vi "LoadFromText.vi"(8 "error in":errorcluster, 9 "String":string, 10 "editor refs":refnum<vi>[](array[refnum]), 11 "Tree ref":refnum<vi>) -> (0 "error out":errorcluster, 3 "Tree ref out":refnum<vi>)   [LabVIEW 2019, in "ScriptManager.lvlib"]
uses:
  ScriptManager.lvlib
  <vilib>/regexp/Match Regular Expression.xnode
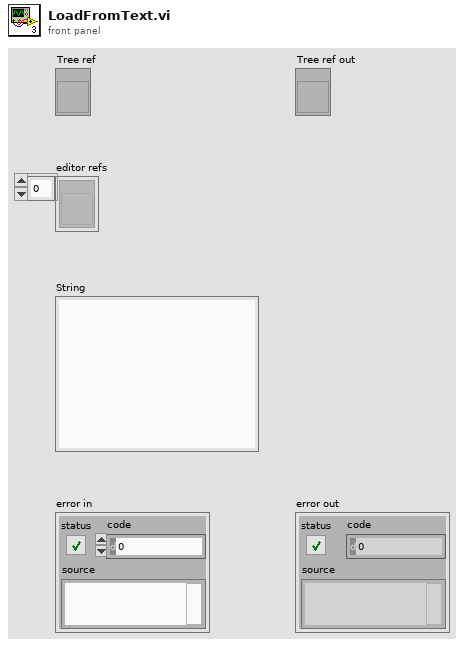
[diagram p1: front panel]
types:
  T1 = cluster{"Left Cell String":string, "Child Text":string[], "Item Indent":i32, "Open?":bool, "Symbol":i32}
  T2 = cluster{"[0]":string, "[1]":string, "[2]":string, "[3]":string, "[4]":string, "[5]":string, "[6]":string, "[7]":string}
  T3 = cluster{"[0]":i32, "[1]":i32, "[2]":i32, "[3]":i32}
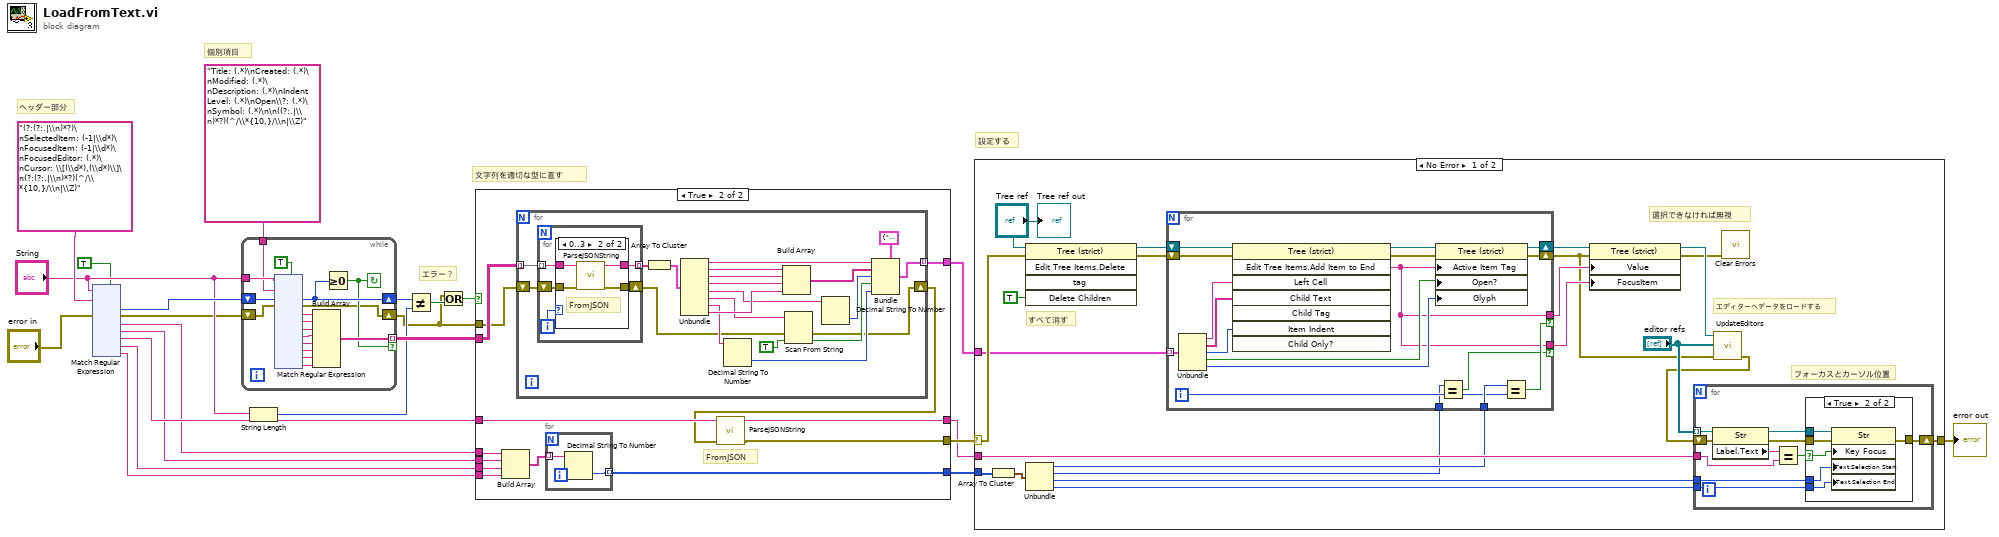
[diagram p0: block diagram]
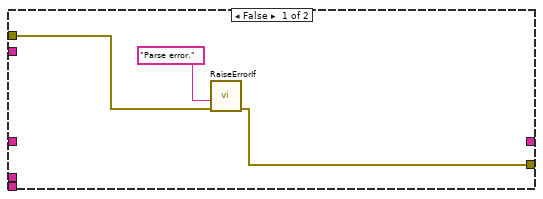
[diagram p4: hidden frame]
diagram:
  # "設定する"
  # "文字列を適切な型に直す"
  # "エラー？"
  # "ヘッダー部分"
  # "個別項目"
  n1 = xnode "Match Regular Expression"("input string"="String", "regular expression"="(?:(?:.|\\n)*?)\nSelectedItem: (-1|\\d*)\nFocusedItem: (-1|\\d*)\nFocusedEditor: (.*)\nCursor: \\[(\\d*),(\\d*)\\]\n(?:(?:.|\\n)*?)(^/\\*{10,}/\\n|\\Z)", "error in"="error in", "multiline? (F)"=TRUE) -> ("offset past match"=w21:i32, "error out"=w14:errorcluster, "submatch 1"=w1:string, "submatch 2"=w2:string, "submatch 3"=w3:string, "submatch 4"=w4:string, "submatch 5"=w5:string)  [unwired: 2 in, 3 out]
  n2 = while {
    tunnel: "String" -> [w40]
    tunnel: "Title: (.*)\nCreated: (.*)\nModified: (.*)\nDescription: (.*)\nIndent Level: (.*)\nOpen\\?: (.*)\nSymbol: (.*)\n\n((?:.|\\n)*?)(^/\\*{10,}/\\n|\\Z)" ("regular expression") -> [w39]
    shift-right: [w36] -> w18
    shift-left: w21 -> [w37]
    tunnel: [w27] -> w22 mode=indexing if=w26
    shift-right: [w24] -> w12
    shift-left: w14 -> [w25]
    stop <- w26 continue-if-true
    n3 = xnode "Match Regular Expression"("input string"=w40, "regular expression"=w39, "offset (0)"=w37, "error in"=w25, "multiline? (F)"=TRUE) -> ("offset past match"=w36:i32, "error out"=w24:errorcluster, "submatch 1"=w35:string, "submatch 2"=w34:string, "submatch 3"=w33:string, "submatch 4"=w32:string, "submatch 5"=w31:string, "submatch 6"=w30:string, "submatch 7"=w29:string, "submatch 8"=w28:string)  [unwired: 1 in, 3 out]
    n4 = Build Array(w35, w34, w33, w32, w31, w30, w29, w28) -> (w27:string[])
    n5 = Greater Or Equal To 0?(x=w36) -> (x >= 0?=w26:bool)
  }
  n6 = String Length(string="String") -> (length=w17:i32)
  n7 = Not Equal?(x=w18, y=w17) -> (x != y?=w16:bool)
  n8 = Or(x=w12, y=w16) -> (x .or. y?=w13:bool)
  n9 = case shown="True" w13 {
    tunnel: w22 -> [_ w182]
    tunnel: w12 -> [w167 w181]
    tunnel: w2 -> [_ w180]
    tunnel: w3 -> [_ w177]
    tunnel: w4 -> [_ w179]
    tunnel: w5 -> [_ w178]
    tunnel: [_ w175] -> w9
    tunnel: [w168 w173] -> w11
    tunnel: [_ w172] -> w8
    tunnel: [_ w171] -> w10
    tunnel: w1 -> [_ w170]
    frame False {
      n10 = call "RaiseErrorIf.vi"("error in (no error)"=w167, "error message"="Parse error.") -> ("error out"=w168:errorcluster)  [unwired: 9 in]
    }
    frame True {
      # "FromJSON"
      n11 = Build Array(w170, w180, w179, w178) -> (w176:string[])
      n12 = for {
        tunnel: w182 -> [w204] mode=indexing
        shift-right: [w186] -> w174
        shift-left: w181 -> [w194]
        tunnel: [w185] -> w171 mode=indexing
        n13 = for {
          tunnel: w204 -> [w210] mode=indexing
          tunnel: [w209] -> w203 mode=indexing
          shift-right: [w206] -> w193
          shift-left: w194 -> [w207]
          i -> [w208]
          n14 = case shown="0..3" w208 {
            tunnel: w210 -> [w212 w216]
            tunnel: [w212 w215] -> w209
            tunnel: w207 -> [w211 w214]
            tunnel: [w211 w213] -> w206
            frame Default {
            }
            frame 0..3 {
              # "FromJSON"
              n15 = call "ParseJSONString.vi"("error in (no error)"=w214, "JSON string"=w216) -> ("error out"=w213:errorcluster, "string"=w215:string)  [unwired: 8 in]
            }
          }
        }
        n16 = Array To Cluster(array=w203) -> (cluster=w205:T2)
        n17 = Unbundle(w205) -> ("[0]"=w191:string, "[1]"=w202:string, "[2]"=w201:string, "[3]"=w200:string, "[4]"=w198:string, "[5]"=w196:string, "[6]"=w197:string, "[7]"=w199:string)
        n18 = Decimal String To Number(string=w197) -> (number=w187:i32)  [unwired: 2 in, 1 out]
        n19 = Build Array(w202, w201, w200, w199) -> (w190:string[])
        n20 = Scan From String(input string=w196, error in=w193, default 1=TRUE) -> (error out=w186:errorcluster, output 1=w188:bool)  [unwired: 2 in, 2 out]
        n21 = Decimal String To Number(string=w198) -> (number=w189:i32)  [unwired: 2 in, 1 out]
        n22 = Bundle(cluster=T1 {"Left Cell String"="", "Child Text"=[], "Item Indent"=0, "Open?"=FALSE, "Symbol"=0}, "Left Cell String"=w191, "Child Text"=w190, "Item Indent"=w189, "Open?"=w188, "Symbol"=w187) -> (w185:T1)
      }
      n23 = for {
        tunnel: w176 -> [w184] mode=indexing
        tunnel: [w183] -> w175 mode=indexing
        n24 = Decimal String To Number(string=w184) -> (number=w183:i32)  [unwired: 2 in, 1 out]
      }
      n25 = call "ParseJSONString.vi"("error in (no error)"=w174, "JSON string"=w177) -> ("error out"=w173:errorcluster, "string"=w172:string)  [unwired: 8 in]
    }
  }
  n26 = case shown="No Error" w11 {
    selector: w11 -> [w236 w274]
    tunnel: w10 -> [w235 _]
    tunnel: w9 -> [w232 _]
    tunnel: w8 -> [w228 _]
    tunnel: [w226 w274] -> w7
    frame No Error {
      # "選択できなければ無視"
      # "フォーカスとカーソル位置"
      # "エディターへデータをロードする"
      # "すべて消す"
      n27 = Array To Cluster(array=w232) -> (cluster=w231:T3)
      n28 = invoke class="Tree (strict)" method="Edit Tree Items.Delete"(reference="Tree ref", error in=w236, "Delete Children"=TRUE ("Delete Children?")) -> (reference out=w234:refnum<vi>, error out=w233:errorcluster)  [unwired: 2 in, 3 out]
      n29 = Unbundle(w231) -> ("[0]"=w225:i32, "[1]"=w220:i32, "[2]"=w221:i32, "[3]"=w222:i32)
      n30 = for {
        tunnel: w235 -> [w271] mode=indexing
        shift-right: [w263] -> w218
        shift-left: w233 -> [w264]
        shift-right: [w262] -> w224
        shift-left: w234 -> [w265]
        tunnel: w225 -> [w261]
        tunnel: [w257] -> w223 if=w260
        tunnel: w220 -> [w258]
        tunnel: [w257] -> w219 if=w256
        i -> [w259]
        n31 = Unbundle(w271) -> ("Left Cell String"=w270:string, "Child Text"=w269:string[], "Item Indent"=w268:i32, "Open?"=w267:bool, "Symbol"=w266:i32)
        n32 = invoke class="Tree (strict)" method="Edit Tree Items.Add Item to End"(reference=w265, error in=w264, "Left Cell"=w270, "Child Text"=w269, "Item Indent"=w268) -> (reference out=w272:refnum<vi>, error out=w273:errorcluster, "Edit Tree Items:Add Item to End"=w257:string)  [unwired: 3 in, 5 out]
        n33 = property class="Tree (strict)"(reference=w272, error in=w273, "Active Item Tag"=w257, "Open?"=w267, "Glyph"=w266) -> (reference out=w262:refnum<vi>, error out=w263:errorcluster)
        n34 = Equal?(x=w258, y=w259) -> (x = y?=w256:bool)
        n35 = Equal?(x=w261, y=w259) -> (x = y?=w260:bool)
      }
      n36 = property class="Tree (strict)"(reference=w224, error in=w218, "Value"=w223, "FocusItem"=w219) -> (reference out=w230:refnum<vi>, error out=w217:errorcluster)
      n37 = call "UpdateEditors.vi"("error in (no error)"=w218, "Array"="editor refs", "TreeControl in"=w230) -> ("error out"=w227:errorcluster)  [unwired: 8 in]
      n38 = for {
        tunnel: "editor refs" -> [w248] mode=indexing
        tunnel: w221 -> [w240]
        tunnel: w222 -> [w239]
        tunnel: w228 -> [w245]
        shift-right: [w241] -> w226
        shift-left: w227 -> [w247]
        n39 = property class="Str"(reference=w248, error in=w247) -> (reference out=w243:refnum<vi>, error out=w242:errorcluster, "Label.Text"=w246:string)
        n40 = Equal?(x=w246, y=w245) -> (x = y?=w244:bool)
        n41 = case shown="True" w244 {
          selector: w244 -> [_ w250]
          tunnel: w243 -> [_ w255]
          tunnel: w242 -> [w249 w254]
          tunnel: [w249 w253] -> w241
          tunnel: w240 -> [_ w251]
          tunnel: w239 -> [_ w252]
          frame False {
          }
          frame True {
            n42 = property class="Str"(reference=w255, error in=w254, "Key Focus"=w250, "Text.Selection Start"=w251, "Text.Selection End"=w252) -> (error out=w253:errorcluster)  [unwired: 1 out]
          }
        }
      }
      n43 = call <vilib>:"Clear Errors.vi"("error in (no error)"=w217) -> ()  [unwired: 5 in, 2 out]
      "Tree ref out" <- "Tree ref"
    }
    frame Error {
    }
  }
  "error out" <- w7
